vi "app_properties.vi"() -> ()   [LabVIEW 2021]
uses:
  <vilib>/Utility/miscctls.llb/LVAllMonitorsDisplayTypeDef.ctl
panel:
  out "Application:Kind":T1(ring)
  out "Display:All Monitors":T2
  out "Application:All VIs In Memory":string[](array[string])
  out "Application:User Name":string
  out "Operating System:Version Number":string
  out "Operating System:Detailed Name":string
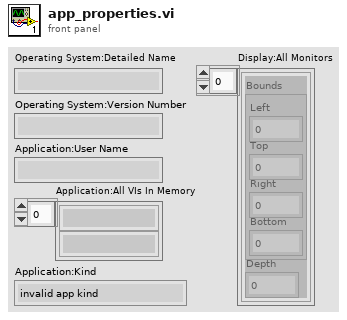
[diagram p1: front panel]
types:
  T1 = enum32{"invalid app kind", "Development System", "Run Time System", "Student Edition", "Embedded LabVIEW", "Evaluation", "Custom"}
  T2 = typedef "LVAllMonitorsDisplayTypeDef.ctl" = cluster{"Bounds":cluster{"Left":i16, "Top":i16, "Right":i16, "Bottom":i16}, "Depth":i16}[]
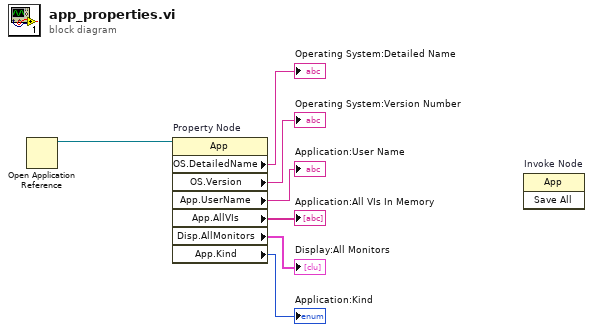
[diagram p0: block diagram]
diagram:
  n1 = Open Application Reference() -> (3:w3:refnum<vi>)  [unwired: 4 in, 1 out]
  n2 = property on="Property Node" class="App"(reference=w3) -> ("OS.DetailedName"=→"Operating System:Detailed Name":string, "OS.Version"=→"Operating System:Version Number":string, "App.UserName"=→"Application:User Name":string, "App.AllVIs"=→"Application:All VIs In Memory":string[], "Disp.AllMonitors"=→"Display:All Monitors":T2, "App.Kind"=→"Application:Kind":T1)  [unwired: 1 in, 2 out]
  n3 = invoke on="Invoke Node" class="App" method="Save All"() -> ()  [unwired: 3 in, 3 out]
